vi "AxisSpace.vi"() -> ()   [LabVIEW 2010]
uses:
  Typedefs/AxisSpaceCfg_ArrayofAxisCfg.ctl
  Typedefs/AxisCfg_cluster.ctl
  <vilib>/Motion/FlexMotion/CustomControls/CustomControls.llb/Axis To Read.flx
panel:
  in  "Axis Space":T1=[{"Axis"=1, "Counts/Rev"=1000.0, "Gear Ratio"=62.6111, "Home Position"=2.6245}, {"Axis"=2, "Counts/Rev"=800.0, "Gear Ratio"=107.815, "Home Position"=2.3132}, {"Axis"=3, "Counts/Rev"=1000.0, "Gear Ratio"=53.7063, "Home Position"=1.8778}, {"Axis"=4, "Counts/Rev"=1000.0, "Gear Ratio"=76.03636, "Home Position"=2.2221}, {"Axis"=5, "Counts/Rev"=1000.0, "Gear Ratio"=71.923, "Home Position"=3.7734}, {"Axis"=6, "Counts/Rev"=1000.0, "Gear Ratio"=76.686, "Home Position"=0.0}] {"Axis" items=["Axis 1"=1, "Axis 2"=2, "Axis 3"=3, "Axis 4"=4, "Axis 5"=5, "Axis 6"=6, "Axis 7"=7, "Axis 8"=8]}
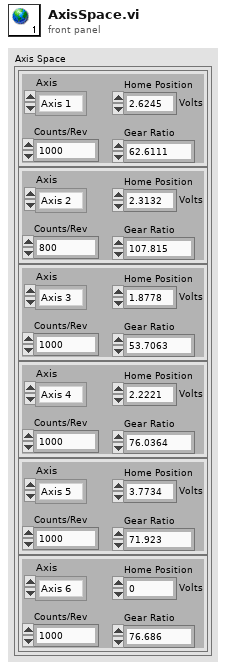
[diagram p1: front panel]
types:
  T1 = typedef "AxisSpaceCfg_ArrayofAxisCfg.ctl" = T2[]
  T2 = typedef "AxisCfg_cluster.ctl" = cluster{"Axis":T3, "Counts/Rev":dbl, "Gear Ratio":dbl, "Home Position":dbl}
  T3 = typedef "Axis To Read.flx" = u16
diagram:
